vi "Registration.vi"(10 "Self Event":refnum<data-value>) -> (0 "error out":errorcluster, 2 "Registration":refnum<event-registration>)   [LabVIEW 2021, in "jettl.lvlib" / "Self Event.lvlib"]
uses:
  Self Event.lvlib
  Msg Strategy/Msg Strategy.lvclass
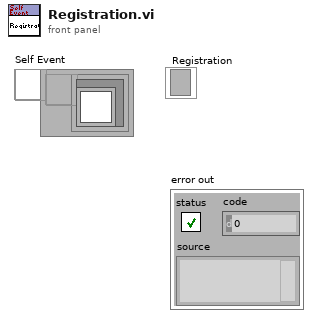
[diagram p1: front panel]
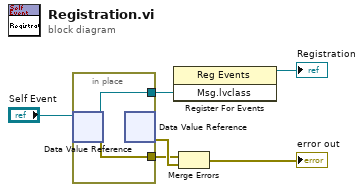
[diagram p0: block diagram]
diagram:
  n1 = in-place {
    in-place-border: [w8] -> w5
    in-place-border: [w7] -> w2
    n2 = in-place-dvr #1("Self Event") -> (w7:refnum<user-event>, w8:errorcluster)
    n3 = in-place-dvr #1() -> (w6:errorcluster)  [unwired: 1 in, 1 out]
  }
  n4 = register-events(w2) -> (reference out=→"Registration":refnum<event-registration>)  [unwired: 2 in, 1 out]
  n5 = Merge Errors(w5, w6) -> (→"error out":errorcluster)
